vi "Test Sync Device.vi"() -> ()   [LabVIEW 2023, in "Application.lvlib"]
uses:
  Application/Application.lvlib
  <vilib>/ActorFramework/Actor/Actor.lvclass
  <vilib>/ActorFramework/Stop Msg/Stop Msg.lvclass
  Sync Device Messages/Start Streaming Msg/Start Streaming Msg.lvclass
  Arduino DQ/Arduino DAQ.lvclass
  Resources/Type Defs/Camera Settings.ctl
panel:
  in  "Camera Settings":T1={"Exposure Time (ms)"=100.0, "Binning"=enum."2x2", "Scan Mode"=-1, "Frames to Acquire"=1000.0, "Pixel Correction"=FALSE, "Frames to Skip"=1, "File Path"=path "", "Duty cycle"=1.0, "ALEX"=FALSE, "Shutter Enable"=[], "fluidics trigger frame"=0, "Bit Depth"=16, "Image Width (px)"=0, "Image Height (px)"=0, "Horizontal Offset (px)"=0, "Vertical Offset (px)"=0} {"Exposure Time (ms)" min=1.0 max=10000.0 step=1.0}
  in  "Duty Cycle":dbl=1.0 min=0.0 max=1.0 step=0.01 format="%.2f"
  in  "Shutter Enable":bool[](array[boolean])=[TRUE, TRUE, TRUE, TRUE]
  in  "Shutter Lines":string[](array[string])=["Dev1/port1/line0", "Dev1/port1/line1", "Dev1/port1/line2", "Dev1/port1/line3"]
  in  "ALEX":bool=TRUE
  in  "Camera Sync Channel":string="Dev1/port2/line7"
  in  "Interval (ms)":dbl=200.0
  in  "stop":bool
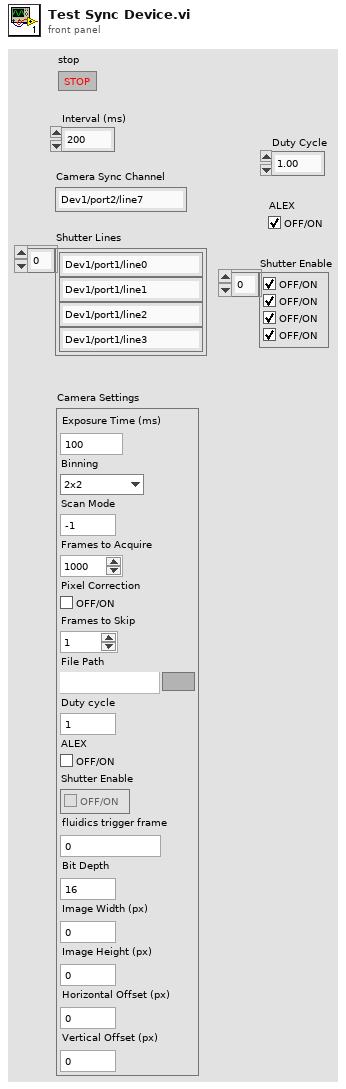
[diagram p1: front panel]
types:
  T1 = typedef "Camera Settings.ctl" = cluster{"Exposure Time (ms)":dbl, "Binning":enum16{"1x1", "2x2", "4x4"}, "Scan Mode":i32, "Frames to Acquire":dbl, "Pixel Correction":bool, "Frames to Skip":u32, "File Path":path, "Duty cycle":dbl, "ALEX":bool, "Shutter Enable":bool[], "fluidics trigger frame":u16, "Bit Depth":u16, "Image Width (px)":u16, "Image Height (px)":u16, "Horizontal Offset (px)":u16, "Vertical Offset (px)":u16}
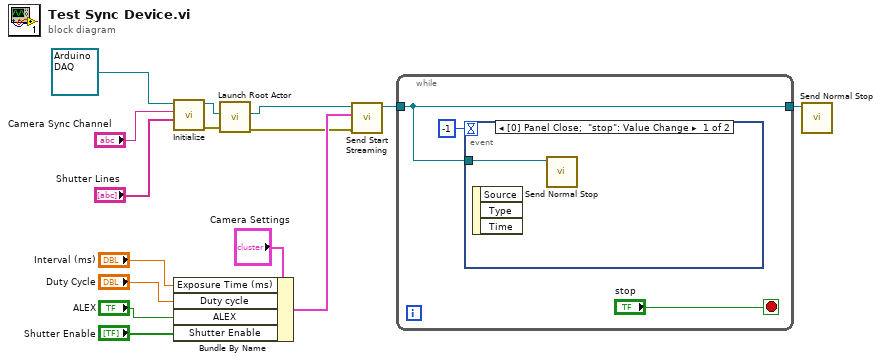
[diagram p0: block diagram]
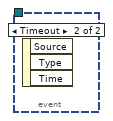
[diagram p2: hidden frame]
diagram:
  n1 = call-dynamic "Initialize.vi"("Shutter Lines"="Shutter Lines", "Sync Line"="Camera Sync Channel", "Synchronization Device in"=refnum<class "Arduino DAQ.lvclass"> refnum ("Arduino DAQ.lvlib:Arduino DAQ.lvclass")) -> ("error out"=w5:errorcluster, "Synchronization Device out"=w4:refnum<class "Arduino DAQ.lvclass">)  [unwired: 7 in]
  n2 = Bundle By Name(cluster="Camera Settings", "Exposure Time (ms)"="Interval (ms)", "Duty cycle"="Duty Cycle", "ALEX"="ALEX", "Shutter Enable"="Shutter Enable") -> (w7:T1)
  n3 = call <vilib>:"Launch Root Actor.vi"("error in (no error)"=w5, "Actor"=w4) -> ("error out"=w6:errorcluster, "Actor's Enqueuer"=w8:refnum<class "Message Enqueuer.lvclass">)  [unwired: 8 in]
  n4 = call "Send Start Streaming.vi"("error in (no error)"=w6, "Camera Settings"=w7, "Message Enqueuer"=w8) -> ("Message Enqueuer out"=w9:refnum<class "Message Enqueuer.lvclass">)  [unwired: 7 in, 1 out]
  n5 = while {
    tunnel: w9 -> [w17]
    tunnel: [w17] -> w15
    stop <- "stop" stop-if-true
    n6 = event shown="[0] Panel Close;  \"stop\": Value Change" {
      selector: _ -> [_ _]
      dyn-events: _ -> [_ _]
      timeout: -1 -> [_ _]
      tunnel: w17 -> [w19 _]
      event Panel Close; "stop": Value Change {
        n7 = event-data() -> ()  [unwired: 1 in, 3 out]
        n8 = call <vilib>:"Send Normal Stop.vi"("Message Enqueuer"=w19) -> ()  [unwired: 10 in, 1 out]
      }
      event Timeout {
        n9 = event-data() -> ()  [unwired: 1 in, 3 out]
      }
    }
  }
  n10 = call <vilib>:"Send Normal Stop.vi"("Message Enqueuer"=w15) -> ()  [unwired: 10 in, 1 out]
